vi "MeasurementHistory_FGV.vi"(8 "Error in":errorcluster) -> (0 "error out":errorcluster)   [LabVIEW 2025, in "Keysight 34461A DMM Measurement.lvlib"]
uses:
  Keysight 34461A DMM Measurement.lvlib
panel:
  in  "Base Table":string[][](array[string])
  in  "Added Row":string[](array[string])
  out "Table Control":string[][](table)
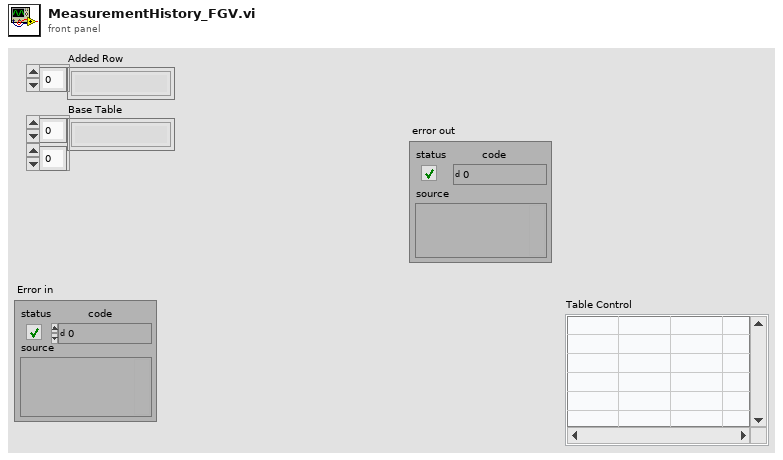
[diagram p1: front panel]
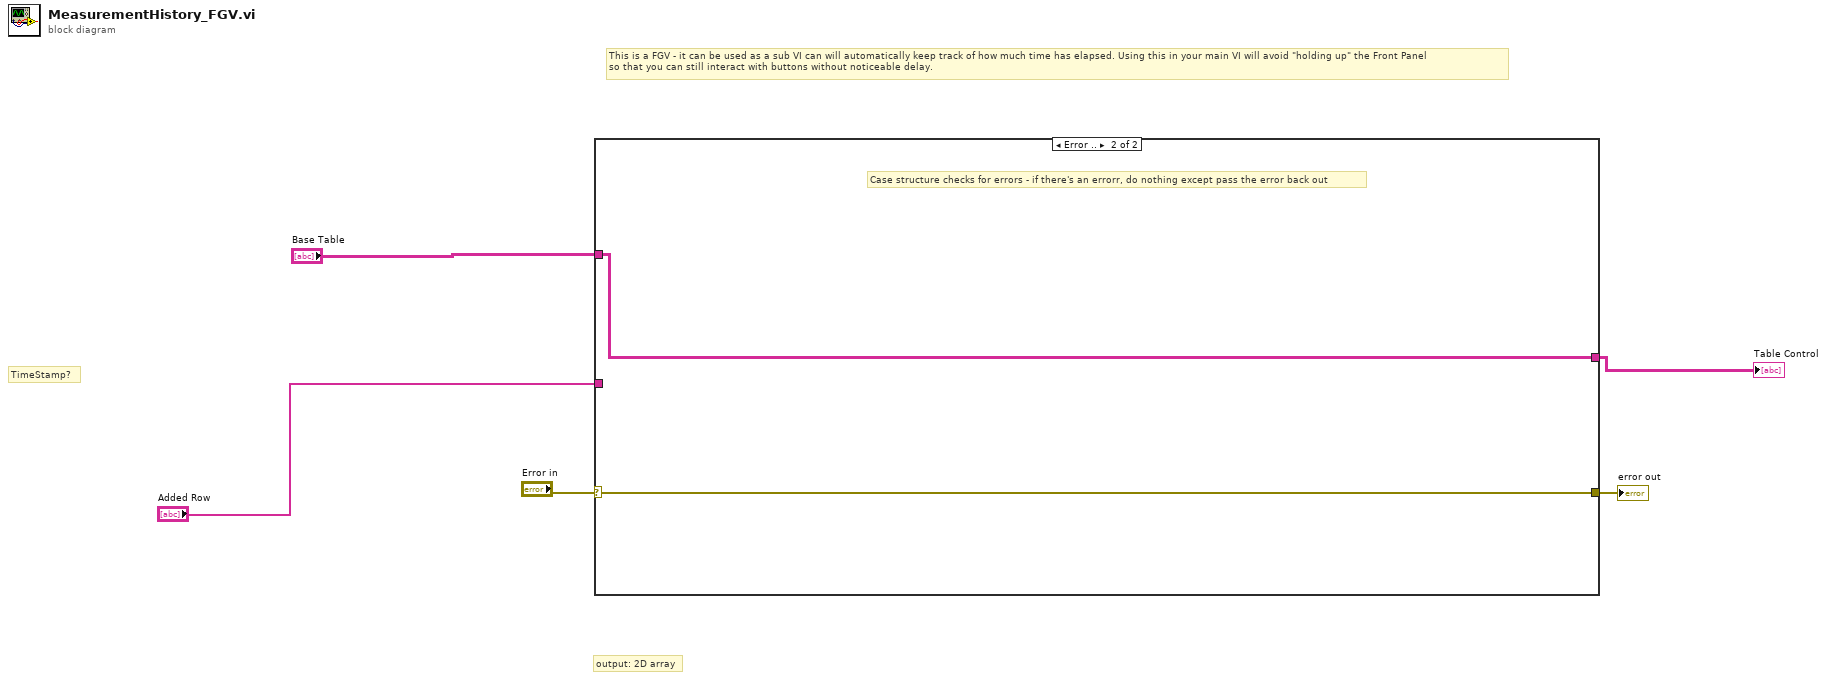
[diagram p0: block diagram]
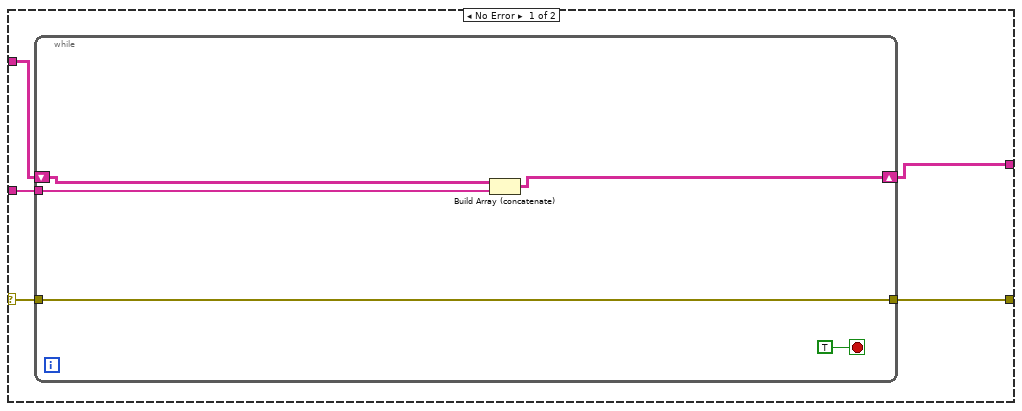
[diagram p2: hidden frame]
diagram:
  # "TimeStamp?"
  # "output: 2D array"
  # "This is a FGV - it can be used as a sub VI can will automatically keep track of how much time has elapsed. Using this in your main VI will avoid \"holding up\" the Front Panel \nso that you can still interact with buttons without noticeable delay."
  n1 = case shown="Error .." "Error in" {
    selector: "Error in" -> [w10 w17]
    tunnel: [w9 w17] -> w4
    tunnel: [w8 w16] -> w1
    tunnel: "Added Row" -> [w7 _]
    tunnel: "Base Table" -> [w6 w16]
    frame No Error {
      n2 = while {
        tunnel: w10 -> [w14]
        tunnel: [w14] -> w9
        shift-right: [w12] -> w8
        shift-left: w6 -> [w13]
        tunnel: w7 -> [w11]
        stop <- TRUE stop-if-true
        n3 = Build Array (concatenate)(w13, w11) -> (w12:string[][])
      }
    }
    frame Error {
      # "Case structure checks for errors - if there's an errorr, do nothing except pass the error back out"
    }
  }
  "error out" <- w4
  "Table Control" <- w1
